vi "RemoveBackgrund1D.vi"(5 "smooth data":bool=TRUE, 7 "Expected FWHM (xy)":dbl=2.2, 11 "Waveform Graph":i32[](graph)=array[5496 elements]) -> (3 "Waveform Graph 3":i32[](graph))   [LabVIEW 2011]
uses:
  <vilib>/Analysis/NI_AALPro.lvlib
panel:
  out "balance parameter 2":dbl=-1.0
  out "Waveform Graph 4":i32[](graph)
  out "balance parameter":dbl=1e-08
  out "Waveform Graph 2":dbl[](graph)
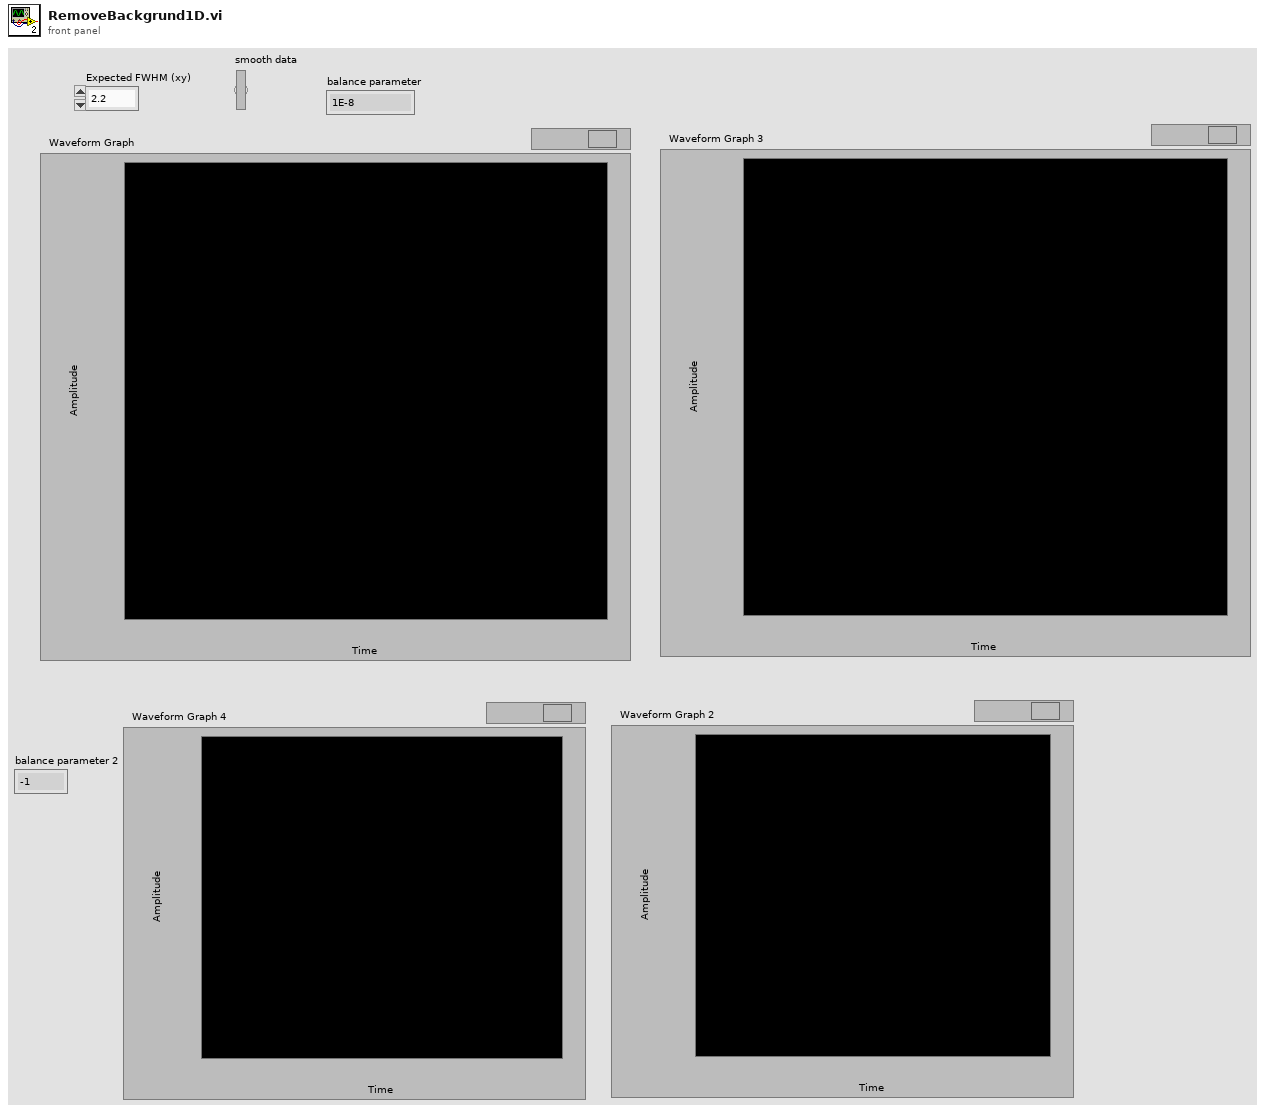
[diagram p1: front panel]
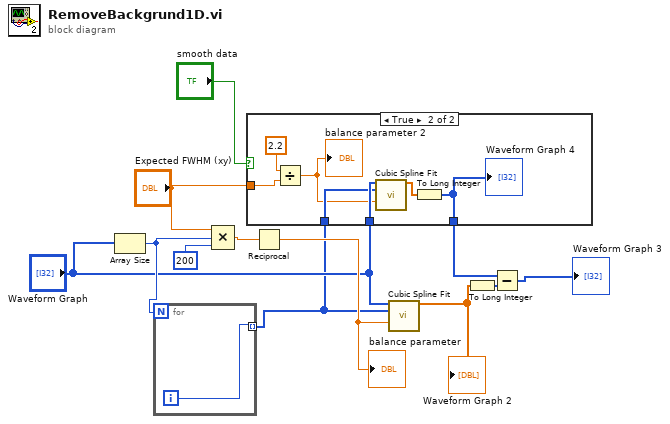
[diagram p0: block diagram]
diagram:
  n1 = Array Size(array="Waveform Graph") -> (size(s)=w12:i32)
  n2 = for {
    N: w12 -> [_]
    tunnel: [w13] -> w5 mode=indexing
    i -> [w13]
  }
  n3 = Compound Arithmetic op=MULTIPLY("Expected FWHM (xy)", w12, 200 ("y")) -> (w9:dbl)
  n4 = case shown="True" "smooth data" {
    tunnel: "Waveform Graph" -> [w14 w21]
    tunnel: w5 -> [_ w20]
    tunnel: "Expected FWHM (xy)" -> [_ w16]
    tunnel: [w14 w18] -> w3
    frame False {
    }
    frame True {
      n5 = Divide(x=2.2, y=w16) -> (x/y=w15:dbl)
      "balance parameter 2" <- w15
      n6 = call <vilib>:"Cubic Spline Fit.vi"("Y"=w21, "X"=w20, "balance parameter"=w15) -> ("Best Cubic Spline Fit"=w19:dbl[])  [unwired: 11 in, 1 out]
      n7 = To Long Integer(number=w19) -> (32bit integer=w18:i32[])
      "Waveform Graph 4" <- w18
    }
  }
  n8 = Reciprocal(x=w9) -> (1/x=w7:dbl)
  "balance parameter" <- w7
  n9 = call <vilib>:"Cubic Spline Fit.vi"("Y"="Waveform Graph", "X"=w5, "balance parameter"=w7) -> ("Best Cubic Spline Fit"=w11:dbl[])  [unwired: 11 in, 1 out]
  "Waveform Graph 2" <- w11
  n10 = To Long Integer(number=w11) -> (32bit integer=w10:i32[])
  n11 = Subtract(x=w3, y=w10) -> (x-y=→"Waveform Graph 3":i32[])
